vi "Dashboard Main.vi"() -> ()   [LabVIEW 2016]
uses:
  <vilib>/Rock Robotics/WPI/Camera/WPI_CameraExposure Values.ctl
  <vilib>/Rock Robotics/WPI/Camera/WPI_CameraWhite Balance Values.ctl
  <vilib>/Rock Robotics/WPI/Camera/WPI_CameraSettings Read MJPG.ctl
  <vilib>/Rock Robotics/WPI/Camera/WPI_CameraImageSize.ctl
  <vilib>/Utility/miscctls.llb/LVRowAndColumnTypeDef.ctl
  <vilib>/event_ctls.llb/eventvkey.ctl
  <vilib>/Rock Robotics/Network Tables/NT Read Numeric Array.vi
  <vilib>/Rock Robotics/Network Tables/NT Write Boolean.vi
  <vilib>/Rock Robotics/WPI/Dashboard/WPI_DashboardLogging Global.vi
  <vilib>/vision/NI_Vision_Development_Module.lvlib
panel:
  in  "Camera Settings Right":T1={"Frame Rate"=30, "Compression"=30, "Size"=1, "DB Camera Config"=FALSE} {"Frame Rate" scale=1.0..30.0; "Compression" scale=100.0..-1.0; "Size" items=["640x480", "320x240", "160x120"]}
  in  "Camera Name Right":string(combo)="No Camera Selection"
  out "Camera Info":cluster{"Mbps LED":bool, "Mbps":dbl, "fps":dbl} {"fps" format="%#.1g"; "Mbps" format="%#.1g"}
  in  "Camera Settings":T1={"Frame Rate"=30, "Compression"=30, "Size"=1, "DB Camera Config"=FALSE} {"Frame Rate" scale=1.0..30.0; "Compression" scale=100.0..-1.0; "Size" items=["640x480", "320x240", "160x120"]}
  in  "TCP":refnum<k5>
  in  "Rec Mode":enum32{"Stop", "Record", "Playback"}(radio)
  out "Robot IP":string
  out "Image Message":string="Timeout in Camera Communications"
  in  "Dashboard Tab":T2(tab)
  in  "New Gyro":bool
  in  "Degrees Rotated":dbl
  in  "NumAcq":dbl
  in  "Forward Time":dbl
  in  "Station":enum16{"1", "2", "3"}(ring)
  in  "OVERRIDE":bool
  in  "Offset":dbl
  out "Reverse":bool
  in  "Degree  Error":dbl=2.0
  in  "Acq Boundary":dbl=15.0
  in  "Target Drive Speed":dbl=-0.5
  in  "Target Pivot Speed":dbl=0.48
  in  "Comp Bot?":bool
  out "Error Value":dbl
  in  "Left Station":bool caption="Left Station?"
  in  "Select Auto":string(combo)="Your Turn"
  out "NT Connection":bool
  out "MotorChart R":cluster{"Numeric":dbl, "Numeric":dbl}(graph)
  out "MotorChart L":cluster{"Numeric":dbl, "Numeric":dbl}(graph)
  out "MotorSliders R":cluster{"MotorSlide1":dbl, "MotorSlide2":dbl} {"MotorSlide2" scale=-1.0..1.0 scale format="%#_2e"; "MotorSlide1" scale=-1.0..1.0 scale format="%#_2e"}
  out "MotorSliders L":cluster{"MotorSlide1":dbl, "MotorSlide2":dbl} {"MotorSlide2" scale=-1.0..1.0 scale format="%#_2e"; "MotorSlide1" scale=-1.0..1.0 scale format="%#_2e"}
  out "Gyro":dbl(knob) scale=0.0..360.0
  out "JS1 Z":dbl(slide) scale=-1.0..1.0 scale format="%#_2e"
  out "JS1 Graph":cluster{"X":dbl, "Y":dbl}[](graph)
  out "JS1 Buttons":T3
  out "JS2 Z":dbl(slide) scale=-1.0..1.0 scale format="%#_2e"
  out "JS2 Graph":cluster{"X":dbl, "Y":dbl}[](graph)
  out "JS2 Buttons":T3
  out "Mode":T4(ring)=enum."Auto Disabled"
  out "Camera Active":bool
  out "Camera Image Right":T5(plugin-control)
  in  "DB/String 9":string
  in  "DB/String 8":string
  in  "DB/String 7":string
  in  "DB/String 6":string
  in  "DB/String 5":string
  in  "DB/String 4":string
  in  "DB/String 3":string
  in  "DB/String 2":string
  in  "DB/String 1":string
  in  "DB/String 0":string
  in  "DB/Slider 0":dbl(slide) scale=0.0..5.0
  in  "DB/Slider 1":dbl(slide) scale=0.0..5.0
  in  "DB/Slider 2":dbl(slide) scale=0.0..5.0
  in  "DB/Slider 3":dbl(slide) scale=0.0..5.0
  out "DB/LED 3":bool
  out "DB/LED 2":bool
  out "DB/LED 1":bool
  out "DB/LED 0":bool
  in  "DB/Button 3":bool
  in  "DB/Button 2":bool
  in  "DB/Button 1":bool
  in  "DB/Button 0":bool caption="New Name"
  out "String":string
  in  "Test Slider":dbl(slide) scale=0.0..100.0 scale format="%#_3g"
  in  "On/Off":bool caption="Solenoid"
  in  "Test Name":u16(ring) items=["Select the test to run..."]
  in  "Test Tree":string(tree)
  in  "Motor":cluster{"Value":dbl, "Enable":bool} {"Value" scale=-1.0..1.0 scale format="%#_3g"}
  out "Progress":T6 {"Test Progress" scale=0.0..100.0}
  in  "Rev/Fwd":cluster{"Forward":bool, "Reverse":bool}
  in  "Test Ring":u16(ring) items=["Monochrome", "Color"]
  out "Cmd Status":string
  in  "Execute Command":bool
  in  "Command Params":string[][](table)
  in  "Command Selection":i32(listbox)
  in  "CheckList":i32(listbox)
  out "Tree":string(tree)
  out "Camera Image":T5(plugin-control)
  out "Background":bool
  in  "Camera Name":string(combo)="No Camera Selection"
  # "HW"
  # "HW"
  # "Joysticks"
  # "Drive Motors"
  # "Front"
  # "Right"
  # "Left"
  # "Back"
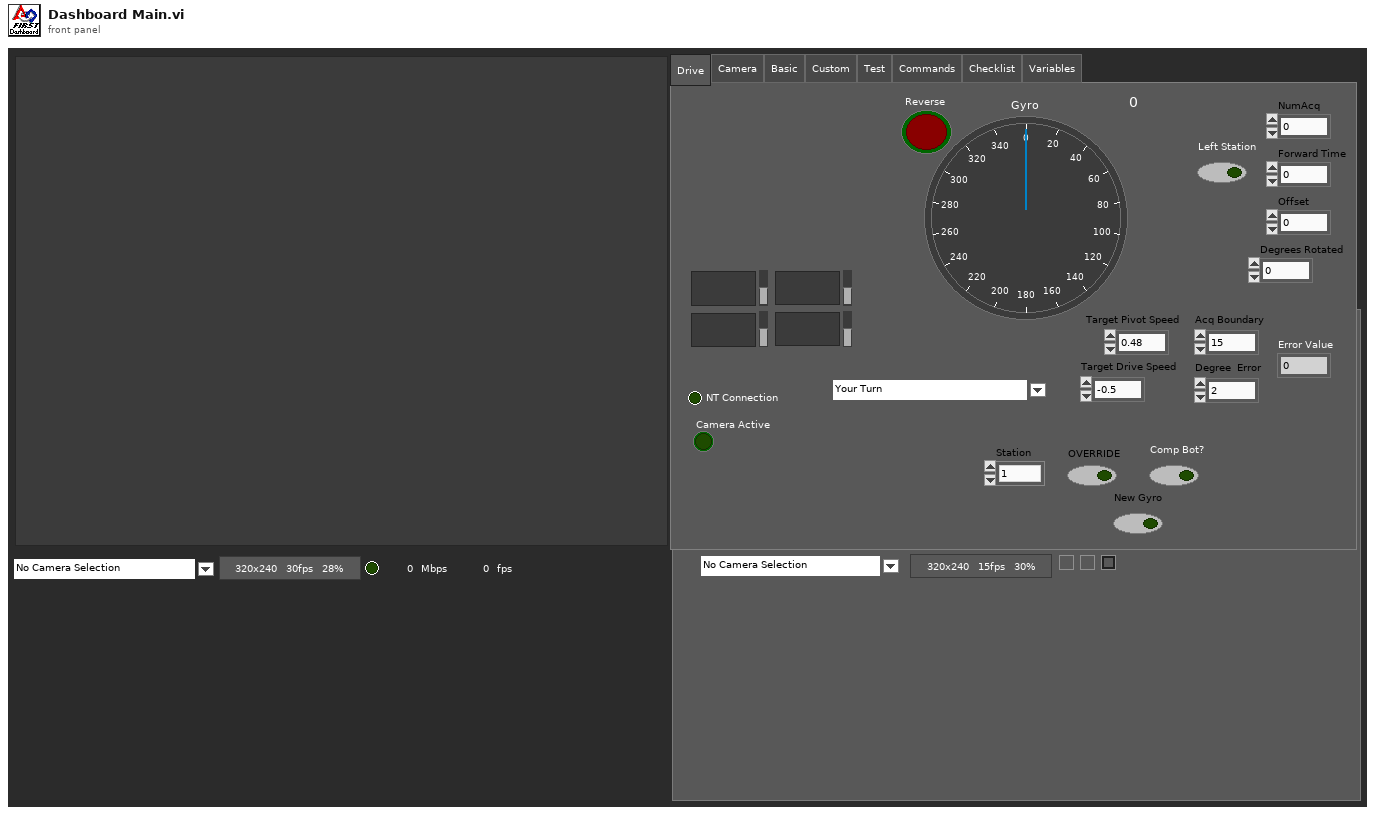
[diagram p1: front panel]
types:
  T1 = cluster{"Frame Rate":i32, "Compression":i32, "Size":u16, "DB Camera Config":bool}
  T2 = enum32{"Drive", "Camera", "Basic", "Custom", "Test", "Commands", "Checklist", "Variables"}
  T3 = cluster{bool, bool, bool, bool, bool, bool, bool, bool, bool, bool, bool, bool}
  T4 = enum8{"Tele-Op Disabled", "Tele-Op Enabled", "Auto Disabled", "Auto Enabled", "Test Disabled", "Test Enabled", "Disconnected", "No Code", "E-Stop"}
  T5 = typedef "IMAQ Image.ctl" = refnum<image>
  T6 = cluster{"Test Progress":u8, "Test Progress Text":string}
  T7 = typedef "Image Type" = u32
  T8 = cluster{"IDs":cluster{"RPC field ID":u16, "Unique ID":u16}, "String":string}
  T9 = enum32{"Drive", "Basic", "Custom", "Test", "Checklist", "Variables"}
  T10 = typedef "WPI_CameraSettings Read MJPG.ctl" = cluster{"fps":i32, "compression":i32, "Image Size":T11, "Config Shown":bool}
  T11 = typedef "WPI_CameraImageSize.ctl" = enum16{"640x480", "320x240", "160x120", "Custom"}
  T12 = typedef "WPI_CameraExposure Values.ctl" = enum16{"Auto", "Flicker-free 50 Hz", "Flicker-free 60 Hz", "Hold current", "Custom"}
  T13 = typedef "WPI_CameraWhite Balance Values.ctl" = enum16{"Auto", "Fixed indoor", "Fixed outdoor 1", "Fixed outdoor 2", "Fixed fluorescent 1", "Fixed fluorescent 2", "Hold current", "Custom"}
  T14 = cluster{"Exposure":T12, "Exposure (%)":dbl, "Brightness":i32, "White Balance":T13, "Color Temp (K)":dbl}
  T15 = cluster{"Brightness":sgl, "Contrast":sgl, "Gamma":sgl}
  T16 = cluster{"Camera Image":refnum<vi>, "Dashboard Tab":refnum<vi>, "Background":refnum<vi>, "Rec Mode":refnum<vi>, "Test Slider":refnum<vi>, "On/Off ":refnum<vi>, "Test Ring":refnum<vi>, "Rev/Fwd":refnum<vi>, "Test Name":refnum<vi>, "Motor":refnum<vi>, "Progress":refnum<vi>, "CheckList":refnum<vi>, "Tree":refnum<vi>, "Test Tree":refnum<vi>, "Command Params":refnum<vi>, "Command Selection":refnum<vi>, "Execute Command":refnum<vi>, "Cmd Status":refnum<vi>, "Camera Settings":refnum<vi>, "Camera Name":refnum<vi>, "Camera Info":refnum<vi>, "Camera Settings Right":refnum<vi>, "Camera Name Right":refnum<vi>, "Camera Image Right":refnum<vi>}
  T17 = cluster{"Error Strings":string, "Disable Counts":cluster{u16, u16}, "Rail Faults":cluster{u16, u16, u16}, "Robot IP":string, "DB Mode":u8, "Event Info":cluster{"Name":string, "Type":u8, "Number":u16, "Replay":u8}}
  T18 = cluster{"Storage":cluster{"Disk Free":u64, "RAM Block":u32, "RAM free":u32}, "CPU Utilization":cluster{"CPU % ISR":sgl, "CPU % Time Crit":sgl, "CPU % Timed Str":sgl, "CPU % High":sgl, "CPU % Above":sgl, "CPU % Normal":sgl, "CPU % Low":sgl}, "CAN":cluster{"% Bus Utilization":sgl, "Bus Off Cnt":u32, "TX_FIFO Full Cnt":u32, "Receive Error Cnt":u8, "Transmit Error Cnt":u8}, "HID":cluster{"HID Outputs":u32, "Rumble Low":u16, "Rumble High":u16}[]}
  T19 = cluster{"Status bits":cluster{"Test Mode":bool, "Autonomous":bool, "Enabled":bool, "Code Start":bool, "Brownout":bool, "Reserved 2":bool, "Reserved 3":bool, "E-Stop":bool}, "Code Trace":cluster{"Disabled":bool, "TeleOp":bool, "Auto":bool, "Test":bool}, "Controller Type":enum16{"unknown", "cRIO", "roboRio"}, "Code?":enum16{"unknown", "noCode", "code"}, "Battery V":dbl}
  T20 = cluster{"Control Bits":cluster{"TestMode":bool, "Autonomous":bool, "Enabled":bool, "FMS Present":bool, bool, bool, bool, "E-Stop":bool}, "Team Station ":u8, "Countdown":sgl, "Joystick Values":cluster{"Axes":dbl[], "Buttons":bool[], "POVs":i16[]}[]}
  T21 = cluster{"Axes":dbl[], "Buttons":bool[], "POVs":i16[]}[]
  T22 = cluster{"Axes":dbl[], "Buttons":bool[], "POVs":i16[]}
  T23 = cluster{"Buttons[0]":bool, "Buttons[1]":bool, "Buttons[2]":bool, "Buttons[3]":bool, "Buttons[4]":bool, "Buttons[5]":bool, "Buttons[6]":bool, "Buttons[7]":bool, "Buttons[8]":bool, "Buttons[9]":bool, "Buttons[10]":bool, "Buttons[11]":bool}
  T24 = cluster{"Operation":enum16{"Update", "Clear"}, "Color Box":u32}[]
  T25 = typedef "eventvkey.ctl" = enum16{"ASCII", "Enter", "Return", "Shift", "Ctrl", "Alt", "Cmd", "Opt", "Caps", "NumLock", "Clear", "Break", "Up", "Down", "Left", "Right", "Insert", "Delete", "Home", "End", "PageUp", "PageDown", "Escape", "Help", "Pause", "ScrollLock", "F1", "F2", "F3", "F4", "F5", "F6", "F7", "F8", "F9", "F10", "F11", "F12", "F13", "F14", "F15", "F16", "F17", "F18", "F19", "F20", "F21", "F22", "F23", "F24", "Play", "VolumeUp", "VolumeDown", "Mute", "Two Byte Char"}
  T26 = cluster{"Image Size":bool, "Image Type":bool, "Pixel Value":bool, "ROI Information":bool, "Zoom Factor":bool}
  T27 = cluster{"Operation":enum16{"Update", "Clear"}, "Color Box":u32}
  T28 = typedef "LVRowAndColumnTypeDef.ctl" = cluster{"Row":i32, "Column":i32}
  T29 = cluster{"Shift":bool, "Ctrl":bool, "Alt":bool, "Cmd":bool, "Opt":bool}
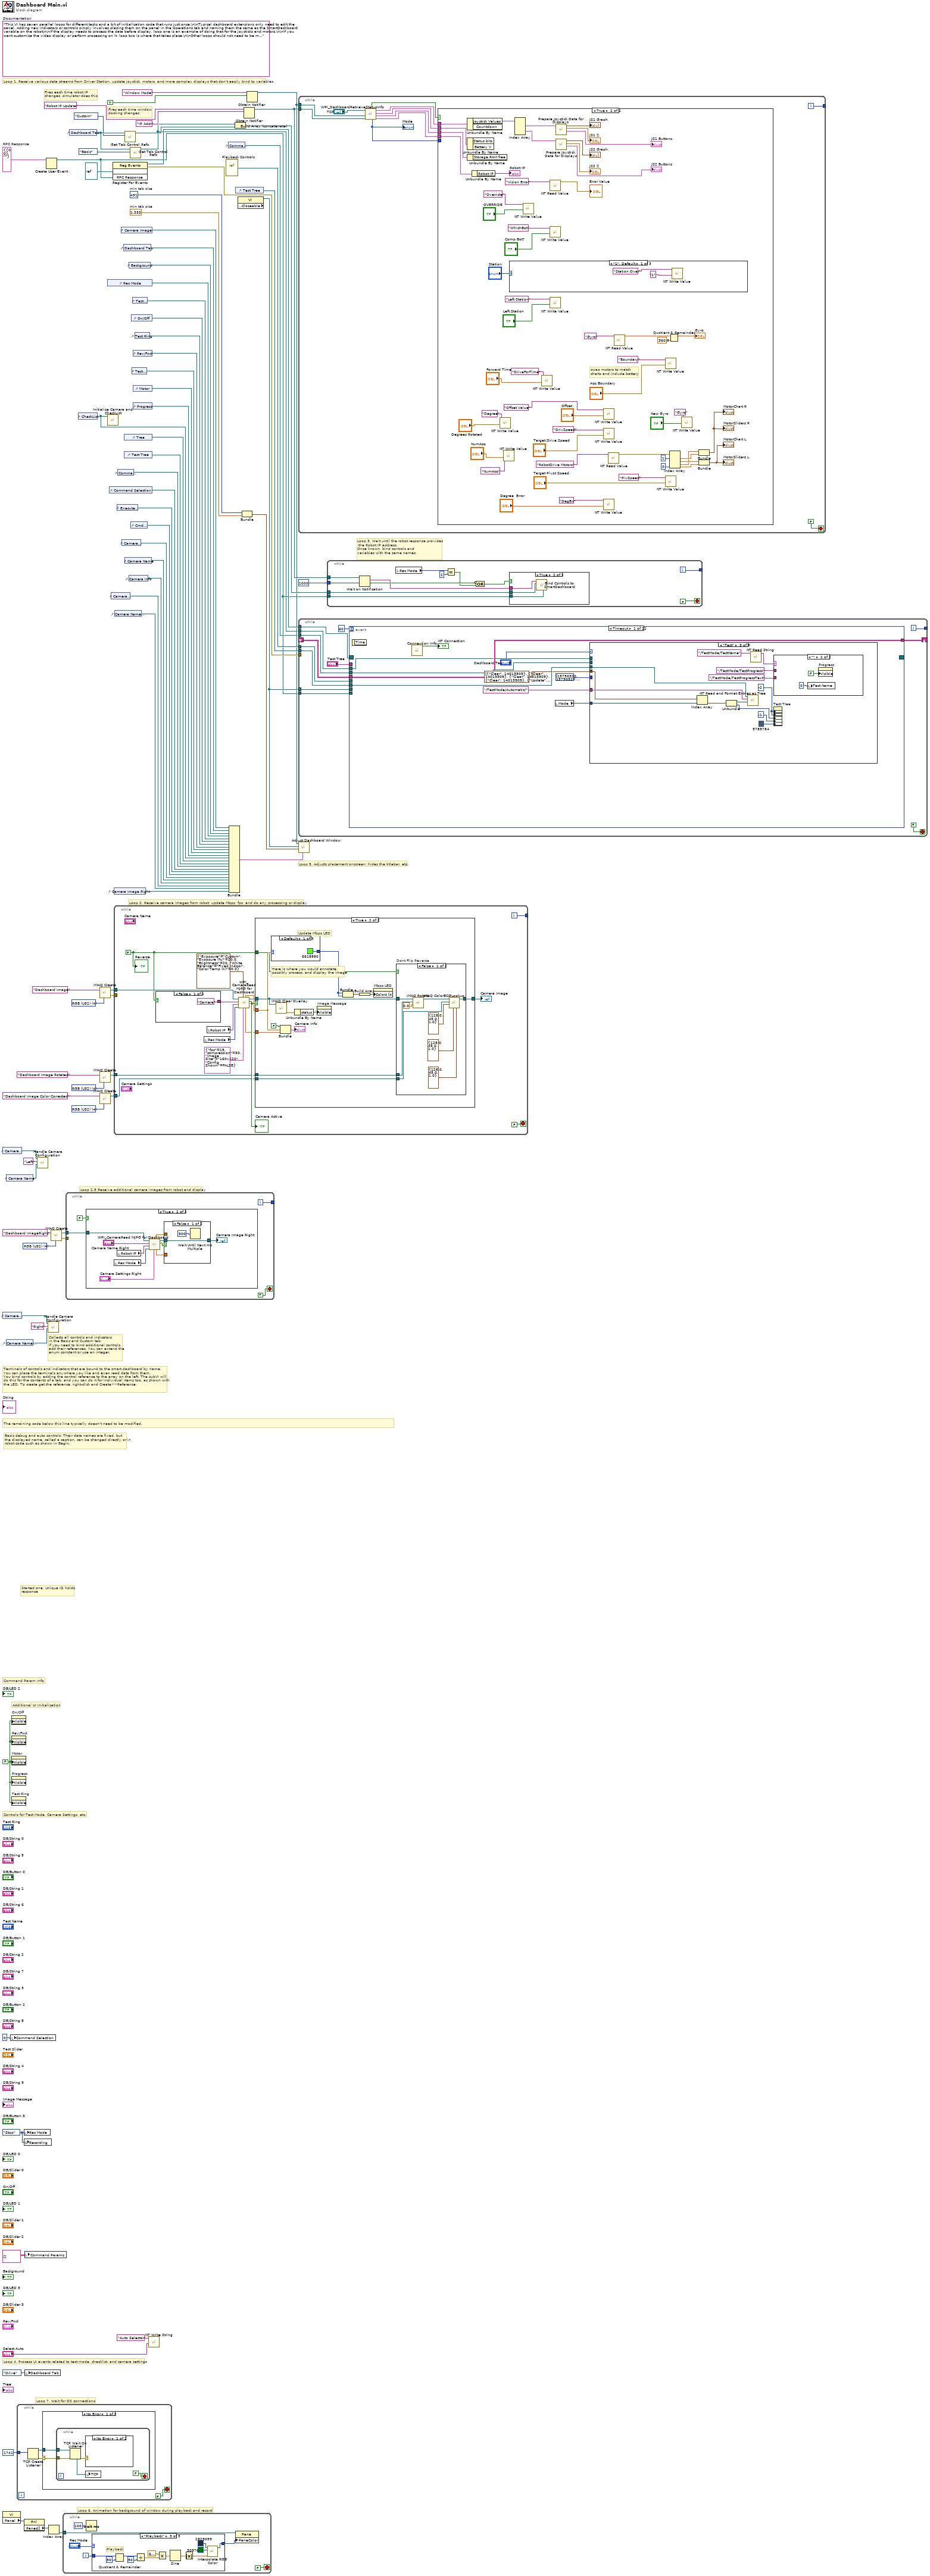
[diagram p0: block diagram]
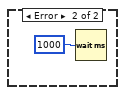
[diagram p4: hidden frame]
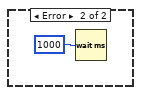
[diagram p5: hidden frame]
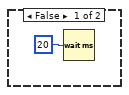
[diagram p6: hidden frame]
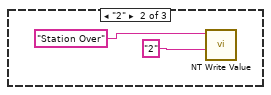
[diagram p7: hidden frame]
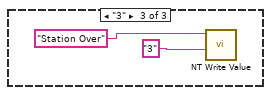
[diagram p8: hidden frame]
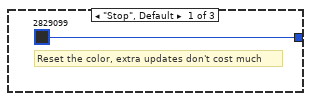
[diagram p9: hidden frame]
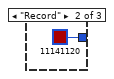
[diagram p10: hidden frame]
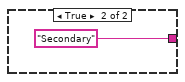
[diagram p12: hidden frame]
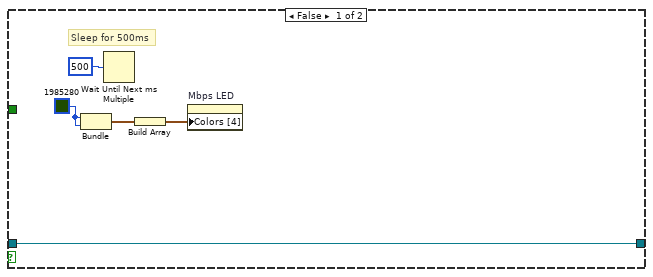
[diagram p13: hidden frame]
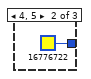
[diagram p15: hidden frame]
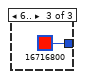
[diagram p16: hidden frame]
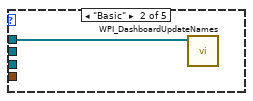
[diagram p18: hidden frame]
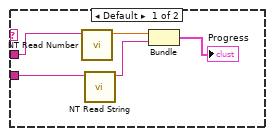
[diagram p19: hidden frame]
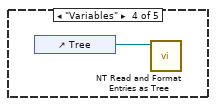
[diagram p20: hidden frame]
diagram:
  w3 = T7 4 items=["Grayscale (U8)", "Grayscale (I16)", "Grayscale (SGL)", "Complex (CSG)", "RGB (U32)", "HSL (U32)", "RGB (U64)"] ("Image Type")
  w6 = T7 4 items=["Grayscale (U8)", "Grayscale (I16)", "Grayscale (SGL)", "Complex (CSG)", "RGB (U32)", "HSL (U32)", "RGB (U64)"] ("Image Type")
  w16 = T7 4 items=["Grayscale (U8)", "Grayscale (I16)", "Grayscale (SGL)", "Complex (CSG)", "RGB (U32)", "HSL (U32)", "RGB (U64)"] ("Image Type")
  w32 = T8 {"IDs"={"RPC field ID"=0, "Unique ID"=0}, "String"=""}  # RPC Response
  w57 = 491  # min tab size
  w56 = 1.333  # min tab size
  w64 = enum32{"Stop", "Record", "Playback"}."Stop" ("Rec Mode")
  w39 = FALSE ("Visible")
  (unwired) "This VI has seven parallel loops for different tasks and a bit of initialization code that runs just once.\n\nTypical dashboard extensions only need to edit the panel. Adding new indicators or controls simply involves placing them on the panel in the Operations tab and naming them the same as the SmartDashboard variable on the robot\n\nIf the display needs to process the data before display, loop one is an example of doing that for the joysticks and motors.\n\nIf you want customize the video display or perform processing on it, loop two is where that takes place.\n\nOther loops should not need to be modified. They are pretty standard, and document the task they perform."  # Documentation
  w81 = T7 4 items=["Grayscale (U8)", "Grayscale (I16)", "Grayscale (SGL)", "Complex (CSG)", "RGB (U32)", "HSL (U32)", "RGB (U64)"] ("Image Type")
  # "Loop 2.5 Receive additional camera images from robot and display"
  # "Command Param Info"
  # "Started one, Unique ID holds\nresponse"
  # "Loop 7. Wait for DS connections"
  # "Basic debug and auto controls: Their data names are fixed, but\nthe displayed name, called a caption, can be changed directly or in\nrobot code such as shown in Begin."
  # "Controls for Test Mode, Camera Settings, etc."
  # "Additional UI Initialization"
  # "Loop 6. Animation for background of window during playback and record"
  # "Fires each time robot IP\nchanges, simulator does this"
  # "Fires each time window\ndocking changes."
  # "Collects all controls and indicators\nin the Basic and Custom tab.\nIf you need to bind additional controls,\nadd their references. You can extend the\nenum constant or use an integer."
  # "The remaining code below this line typically doesn't need to be modified."
  # "Loop 4. Process UI events related to test mode, checklist, and camera settings"
  # "Terminals of controls and indicators that are bound to the smart dashboard by name.\nYou can place the terminals anywhere you like and even read data from them.\nYou bind controls by adding the control reference to the array on the left. The subVI will\ndo this for the contents of a tab, and you can do it for individual items too, as shown with\nthe LED. To create get the reference, right-click and Create>>Reference."
  # "Loop 3. Wait until the robot response provides\n the Robot IP address.\nOnce known, bind controls and\nvariables with the same names."
  # "Loop 5. Adjusts placement onscreen, hides the titlebar, etc."
  # "Loop 1. Receive various data streams from Driver Station, update joystick, motors, and more complex displays that don't easily bind to variables."
  # "Loop 2. Receive camera images from robot, update Mbps, fps, and do any processing or display"
  n1 = control-ref of="Camera Settings"() -> (w25:refnum<vi>)
  n2 = control-ref of="Camera Settings Right"() -> (w13:refnum<vi>)
  n3 = property class="VI"() -> ("Panel"=w71:refnum<vi>)  [unwired: 2 in, 2 out]
  n4 = control-ref of="Camera Name"() -> (w24:refnum<vi>)
  n5 = control-ref of="Camera Name Right"() -> (w12:refnum<vi>)
  n6 = local write "Command Selection"(u16 0 ("milliseconds to wait")) -> ()
  n7 = property on="On/Off" class="Bool (strict)"("Visible"=w39) -> ()  [unwired: 2 in, 2 out]
  n8 = property on="Rev/Fwd" class="Clust (strict)"("Visible"=w39) -> ()  [unwired: 2 in, 2 out]
  n9 = property on="Motor" class="Clust (strict)"("Visible"=w39) -> ()  [unwired: 2 in, 2 out]
  n10 = property on="Progress" class="Clust (strict)"("Visible"=w39) -> ()  [unwired: 2 in, 2 out]
  n11 = property on="Test Ring" class="Ring (strict)"("Visible"=w39) -> ()  [unwired: 2 in, 2 out]
  n12 = while {
    tunnel: u16 1741 ("timeout ms (25000)") -> [w83]
    stop <- FALSE stop-if-true
    n13 = TCP Create Listener(10:w83) -> (0:w82:errorcluster, 3:w84:refnum<k5>)  [unwired: 4 in, 1 out]
    n14 = case shown="No Error" w82 {
      selector: w82 -> [w86 _]
      tunnel: w84 -> [w87 _]
      frame No Error {
        n15 = while {
          tunnel: w87 -> [w90]
          tunnel: w86 -> [w89]
          stop <- FALSE stop-if-true
          n16 = TCP Wait On Listener(8:w89, 11:w90) -> (0:w91:errorcluster, 4:w92:refnum<k5>)  [unwired: 2 in, 3 out]
          n17 = case shown="No Error" w91 {
            frame No Error {
            }
            frame Error {
              n18 = Wait (ms)(milliseconds to wait=u32 1000) -> ()  [unwired: 1 out]
            }
          }
          n19 = local write "TCP"(w92) -> ()
        }
      }
      frame Error {
        n20 = Wait (ms)(milliseconds to wait=u32 1000) -> ()  [unwired: 1 out]
      }
    }
  }
  n21 = local write "Rec Mode"(w64) -> ()
  n22 = global write "WPI_DashboardLogging Global.vi" "Recording"(w64) -> ()
  n23 = property class="Pnl"(reference=w71) -> ("Panes[]"=w72:refnum<vi>[])  [unwired: 1 in, 2 out]
  n24 = local write "Command Params"(string[][] [] ("Command Params")) -> ()
  n25 = local write "Dashboard Tab"(T2."Drive" ("Dashboard Tab")) -> ()
  n26 = call "Handle Camera Configuration.vi"("CameraNameRef"=w24, "Camera File Name"="Left", "ClusterRef"=w25) -> ()  [unwired: 9 in]
  n27 = Create User Event(user event datatype=w32) -> (user event=w28:refnum<user-event>)  [unwired: 1 in, 1 out]
  n28 = call "Handle Camera Configuration.vi"("CameraNameRef"=w12, "Camera File Name"="Right", "ClusterRef"=w13) -> ()  [unwired: 9 in]
  n29 = Index Array(array=w72) -> (element=w70:refnum<vi>)  [unwired: 1 in]
  n30 = call "IMAQ Create"("Image Name"="Dashboard ImageRight", "Image Type"=w16) -> ("New Image"=w15:T5, "error out"=w14:errorcluster)  [unwired: 2 in, 1 out]
  n31 = while {
    tunnel: w70 -> [w96]
    i -> [w99]
    stop <- FALSE stop-if-true
    n32 = Wait (ms)(milliseconds to wait=u32 100) -> ()  [unwired: 1 out]
    n33 = case shown="\"Playback\"" "Rec Mode" {
      tunnel: w99 -> [_ _ w114]
      tunnel: [u32 2829099 ("Base Color") u32 11141120 ("Target Color") w103] -> w95
      frame "Stop", Default {
        # "Reset the color, extra updates don't cost much"
      }
      frame "Record" {
      }
      frame "Playback" {
        # "Playback"
        n34 = Quotient & Remainder(x=w114, y=u32 50 ("milliseconds to wait")) -> (x-y*floor(x/y)=w110:u32)  [unwired: 1 out]
        n35 = Divide(x=w110, y=u32 50 ("milliseconds to wait")) -> (x/y=w107:dbl)
        n36 = Multiply(x=6.283185307179586, y=w107) -> (x*y=w112:dbl)
        n37 = Sine(x=w112) -> (sin(x)=w111:dbl)
        n38 = Absolute Value(x=w111) -> (abs(x)=w104:dbl)
        n39 = call "Interpolate RGB Color.vi"("Proportion"=w104, "Target Color"=u32 30976, "Base Color"=u32 2829099) -> ("Result Color"=w103:u32)  [unwired: 8 in]
      }
    }
    n40 = property class="Pane"(reference=w96, "PaneColor"=w95) -> ()  [unwired: 1 in, 2 out]
  }
  n41 = while {
    tunnel: w15 -> [w118]
    tunnel: w14 -> [_]
    tunnel: [w117] -> _
    i -> [w117]
    stop <- TRUE stop-if-true
    n42 = case shown="True" FALSE {
      tunnel: w118 -> [_ w127]
      frame False {
      }
      frame True {
        n43 = local read "Rec Mode"() -> (w125:enum32{"Stop", "Record", "Playback"})
        n44 = local read "Robot IP"() -> (w126:string)
        n45 = call <vilib>:"WPI_CameraRead MJPG for Dashboard.vi"("Camera Settings"="Camera Settings Right", "Rec Mode"=w125, "Robot IP"=w126, "Camera Name"="Camera Name Right", "Refnum in"=w127) -> ("Active"=w122:bool, "Refnum out"=w123:T5, "FPS"=w120:dbl, "Bandwidth (Mbps)"=w121:dbl)  [unwired: 3 in]
        n46 = case shown="False" w122 {
          tunnel: w123 -> [w129 w131]
          tunnel: w121 -> [_ _]
          tunnel: w120 -> [_ _]
          tunnel: [w129 w131] -> w119
          frame False {
            n47 = Wait Until Next ms Multiple(millisecond multiple=u32 500) -> ()  [unwired: 1 out]
          }
          frame True {
          }
        }
        "Camera Image Right" <- w119
      }
    }
  }
  n48 = control-ref of="Dashboard Tab"() -> (w62:refnum<vi>)
  n49 = control-ref of="CheckList"() -> (w50:refnum<vi>)
  n50 = call "IMAQ Create"("Image Name"="Dashboard Image", "Image Type"=w81) -> ("New Image"=w79:T5, "error out"=w78:errorcluster)  [unwired: 2 in, 1 out]
  n51 = call "IMAQ Create"("Image Name"="Dashboard Image Rotated", "Image Type"=w6) -> ("New Image"=w4:T5)  [unwired: 2 in, 2 out]
  n52 = call "IMAQ Create"("Image Name"="Dashboard Image Color Corrected", "Image Type"=w3) -> ("New Image"=w1:T5)  [unwired: 2 in, 2 out]
  n53 = control-ref of="Rec Mode"() -> (w45:refnum<vi>)
  n54 = call "Initialize Camera and CheckList.vi"("ListBox in"=w50) -> ()  [unwired: 11 in]
  n55 = control-ref of="Command Selection"() -> (w31:refnum<vi>)
  n56 = control-ref of="Camera Settings Right"() -> (w9:refnum<vi>)
  n57 = register-events(refnum<vi> refnum, w28) -> (reference out=w68:refnum<event-registration>, error out=w67:errorcluster)  [unwired: 2 in]
  n58 = control-ref of="Camera Image Right"() -> (w7:refnum<vi>)
  n59 = while {
    tunnel: w79 -> [w145]
    tunnel: w78 -> [_]
    tunnel: [w146] -> _
    tunnel: w4 -> [w137]
    tunnel: w1 -> [w136]
    i -> [w146]
    stop <- FALSE stop-if-true
    w132 = FALSE ("Default Value")
    n60 = case shown="False" w132 {
      tunnel: ["Camera" "Secondary"] -> w135
      frame False {
      }
      frame True {
      }
    }
    n61 = local read "Rec Mode"() -> (w141:enum32{"Stop", "Record", "Playback"})
    n62 = local read "Robot IP"() -> (w140:string)
    n63 = call <vilib>:"WPI_CameraRead MJPG for Dashboard.vi"("Camera Settings"=T10 {"fps"=15, "compression"=30, "Image Size"=enum."160x120", "Config Shown"=FALSE}, "Camera Settings 2"=T14 {"Exposure"=enum."Custom", "Exposure (%)"=20.0, "Brightness"=20, "White Balance"=enum."Fixed indoor", "Color Temp (K)"=0.0}, "Rec Mode"=w141, "Robot IP"=w140, "Camera Name"=w135, "Refnum in"=w145) -> ("Active"=w143:bool, "Refnum out"=w144:T5, "FPS"=w142:dbl, "Bandwidth (Mbps)"=w139:dbl)  [unwired: 2 in]
    "Camera Active" <- w143
    n64 = case shown="True" w143 {
      tunnel: w144 -> [w150 w159]
      tunnel: w139 -> [_ w162]
      tunnel: w142 -> [_ w163]
      tunnel: [w150 w155] -> w138
      tunnel: w137 -> [_ w158]
      tunnel: w136 -> [_ w156]
      tunnel: w132 -> [_ w157]
      frame False {
        w152 = u32 1985280 ("Color Box")
        # "Sleep for 500ms"
        n65 = Bundle("Color Box"=w152, "Color Box"=w152) -> (w153:cluster{"Color Box":u32, "Color Box":u32})  [unwired: 1 out]
        n66 = Wait Until Next ms Multiple(millisecond multiple=u32 500) -> ()  [unwired: 1 out]
        n67 = Build Array(w153) -> (w151:cluster{"Color Box":u32, "Color Box":u32}[])
        n68 = property on="Mbps LED" class="Bool (strict)"("Colors [4]"=w151) -> ()  [unwired: 2 in, 2 out]
      }
      frame True {
        # "Here is where you would annotate,\npossibly process, and display the image"
        # "Update Mbps LED"
        n69 = case shown="Default" w162 {
          tunnel: [u32 6618880 ("Color Box") u32 16776722 ("Color Box") u32 16716800 ("Color Box")] -> w165
          frame Default {
          }
          frame 4, 5 {
          }
          frame 6.. {
          }
        }
        n70 = call "IMAQ Clear Overlay"("Image"=w159) -> ("error out"=w167:errorcluster)  [unwired: 2 in, 8 out]
        n71 = Bundle(FALSE, "Bandwidth (Mbps)"=w162, "FPS"=w163) -> (→"Camera Info":cluster{bool, "Bandwidth (Mbps)":dbl, "FPS":dbl})  [unwired: 1 in]
        n72 = Unbundle By Name(w167) -> ("status"=w168:bool)
        n73 = property on="Image Message" class="Str"("Visible"=w168) -> ()  [unwired: 2 in, 2 out]
        n74 = Bundle("Color Box"=w165, "Color Box"=w165) -> (w166:cluster{"Color Box":u32, "Color Box":u32})  [unwired: 1 out]
        n75 = Build Array(w166) -> (w164:cluster{"Color Box":u32, "Color Box":u32}[])
        n76 = property on="Mbps LED" class="Bool (strict)"("Colors [4]"=w164) -> ()  [unwired: 2 in, 2 out]
        n77 = case "Dont Flip Reverse" shown="False" w157 {
          tunnel: w159 -> [w176 w178]
          tunnel: w158 -> [w175 _]
          tunnel: w156 -> [w171 _]
          tunnel: [w169 w178] -> w155
          frame False {
            n78 = call "IMAQ Rotate"("Angle (degrees)"=sgl 0.0, "Image Dst"=w175, "Image Src"=w176) -> ("Image Dst Out"=w170:T5)  [unwired: 7 in, 1 out]
            n79 = call "IMAQ ColorBCGLookup"("Blue BCG Values"=T15 {"Brightness"=128.0, "Contrast"=45.0, "Gamma"=1.0}, "Green BCG Values"=T15 {"Brightness"=128.0, "Contrast"=45.0, "Gamma"=1.0}, "Red BCG Values"=T15 {"Brightness"=128.0, "Contrast"=45.0, "Gamma"=1.0}, "Image Dst"=w171, "Image Src"=w170) -> ("Image Dst Out"=w169:T5)  [unwired: 5 in, 1 out]
          }
          frame True {
          }
        }
      }
    }
    "Camera Image" <- w138
    "Reverse" <- w132
  }
  n80 = control-ref of="Camera Name Right"() -> (w8:refnum<vi>)
  n81 = control-ref of="Execute Command"() -> (w33:refnum<vi>)
  n82 = control-ref of="Command Params"() -> (w34:refnum<vi>)
  n83 = control-ref of="Camera Image"() -> (w59:refnum<vi>)
  n84 = control-ref of="Camera Settings"() -> (w23:refnum<vi>)
  n85 = control-ref of="Dashboard Tab"() -> (w58:refnum<vi>)
  n86 = control-ref of="Tree"() -> (w49:refnum<vi>)
  n87 = control-ref of="Test Tree"() -> (w48:refnum<vi>)
  n88 = call <vilib>:"Get Tab Control Refs.vi"("Page Index"=T9."Custom" ("Dashboard Tab"), "TabControl in"=w62) -> ("ControlsOnPage"=w61:refnum<vi>[])  [unwired: 9 in]
  n89 = control-ref of="Camera Name"() -> (w22:refnum<vi>)
  n90 = control-ref of="Background"() -> (w54:refnum<vi>)
  n91 = control-ref of="Camera Info"() -> (w21:refnum<vi>)
  n92 = call <vilib>:"Get Tab Control Refs.vi"("Page Index"=T9."Basic" ("Dashboard Tab"), "TabControl in"=w62) -> ("ControlsOnPage"=w20:refnum<vi>[])  [unwired: 9 in]
  n93 = control-ref of="Cmd Status"() -> (w27:refnum<vi>)
  n94 = control-ref of="On/Off"() -> (w43:refnum<vi>)
  n95 = control-ref of="Test Name"() -> (w47:refnum<vi>)
  n96 = control-ref of="Test Slider"() -> (w44:refnum<vi>)
  n97 = control-ref of="Rev/Fwd"() -> (w41:refnum<vi>)
  n98 = control-ref of="Motor"() -> (w46:refnum<vi>)
  n99 = control-ref of="Progress"() -> (w40:refnum<vi>)
  n100 = control-ref of="Test Ring"() -> (w42:refnum<vi>)
  n101 = call <vilib>:"NT Write String.vi"("String"="Select Auto", "Name"="Auto Selector") -> ()  [unwired: 9 in, 1 out]
  n102 = vi-ref "Playback Controls.vi"() -> (w69:refnum<vi>)
  n103 = control-ref of="Command Params"() -> (w26:refnum<vi>)
  n104 = Bundle("Camera Image"=w59, "Dashboard Tab"=w58, "Background"=w54, "Rec Mode"=w45, "Test Slider"=w44, "On/Off"=w43, "Test Ring"=w42, "Rev/Fwd"=w41, "Test Name"=w47, "Motor"=w46, "Progress"=w40, "CheckList"=w50, "Tree"=w49, "Test Tree"=w48, "Command Params"=w34, "Command Selection"=w31, "Execute Command"=w33, "Cmd Status"=w27, "Camera Settings"=w23, "Camera Name"=w22, "Camera Info"=w21, "Camera Settings Right"=w9, "Camera Name Right"=w8, "Camera Image Right"=w7) -> (w51:T16)  [unwired: 1 in]
  n105 = Build Array (concatenate)(w20, w61) -> (w60:refnum<vi>[])
  n106 = control-ref of="Test Tree"() -> (w73:refnum<vi>)
  n107 = property class="VI" props=["Front Panel.Closeable"]() -> (reference out=w63:refnum<vi>)  [unwired: 2 in, 2 out]
  n108 = Bundle("min tab size"=w57, "min tab size"=w56) -> (w55:cluster{"min tab size":i32, "min tab size":dbl})  [unwired: 1 in]
  n109 = Obtain Notifier(name (unnamed)="Robot IP Update", notification data type="IP Addr" ("name (unnamed)")) -> (notifier out=w38:refnum<notifier>)  [unwired: 2 in, 2 out]
  n110 = Obtain Notifier(name (unnamed)="Window Mode", notification data type=TRUE) -> (notifier out=w37:refnum<notifier>)  [unwired: 2 in, 2 out]
  n111 = while {
    tunnel: [w191] -> _
    tunnel: w38 -> [w185]
    tunnel: w37 -> [w182]
    i -> [w191]
    stop <- FALSE stop-if-true
    n112 = call <vilib>:"WPI_DashboardRetrieveStatusInfo.vi"("Binding Refnum"=w185, "Window Mode Notifier"=w182, "TCP Cnx"="TCP") -> ("Power and Errors"=w186:T17, "Robot Metrics"=w189:T18, "Status Info"=w190:T19, "Control Info"=w187:T20, "Robot Mode"=w184:T4, "Process?"=w188:bool)  [unwired: 3 in]
    "Mode" <- w184
    n113 = case shown="True" w188 {
      tunnel: w190 -> [_ w248]
      tunnel: w189 -> [_ w247]
      tunnel: w187 -> [_ w246]
      tunnel: w186 -> [_ w245]
      tunnel: w184 -> [_ _]
      frame False {
        n114 = Wait (ms)(milliseconds to wait=u32 20) -> ()  [unwired: 1 out]
      }
      frame True {
        # "swap motors to match\ncharts and include battery"
        n115 = Unbundle By Name(w246) -> ("Joystick Values"=w236:T21)  [unwired: 1 out]
        n116 = Unbundle By Name(w248) -> ()  [unwired: 2 out]
        n117 = Unbundle By Name(w247) -> ()  [unwired: 1 out]
        n118 = Unbundle By Name(w245) -> ("Robot IP"=→"Robot IP":string)
        n119 = call-poly <vilib>:"NT Write Value.vi"("Numeric"="Degrees Rotated", "Name"="Degree") -> ()  [unwired: 9 in, 1 out]
        n120 = call-poly <vilib>:"NT Write Value.vi"("Numeric"="NumAcq", "Name"="NumAcq") -> ()  [unwired: 9 in, 1 out]
        n121 = case shown="\"1\", Default" "Station" {
          frame "1", Default {
            n122 = call-poly <vilib>:"NT Write Value.vi"("String"="1", "Name"="Station Over") -> ()  [unwired: 9 in, 1 out]
          }
          frame "2" {
            n123 = call-poly <vilib>:"NT Write Value.vi"("String"="2", "Name"="Station Over") -> ()  [unwired: 9 in, 1 out]
          }
          frame "3" {
            n124 = call-poly <vilib>:"NT Write Value.vi"("String"="3", "Name"="Station Over") -> ()  [unwired: 9 in, 1 out]
          }
        }
        n125 = Index Array(array=w236) -> (element #1=w235:T22, element #3=w221:T22)  [unwired: 4 in, 2 out]
        n126 = call-poly <vilib>:"NT Write Value.vi"("Boolean"="OVERRIDE", "Name"="Override") -> ()  [unwired: 9 in, 1 out]
        n127 = call-poly <vilib>:"NT Write Value.vi"("Numeric"="Forward Time", "Name"="DriveForTime") -> ()  [unwired: 9 in, 1 out]
        n128 = call-poly <vilib>:"NT Read Value.vi"("Name"="Vision Error") -> ("Numeric"=→"Error Value":dbl)  [unwired: 9 in, 1 out]
        n129 = call-poly <vilib>:"NT Write Value.vi"("Boolean"="Comp Bot?", "Name"="WhichBot") -> ()  [unwired: 9 in, 1 out]
        n130 = call-poly <vilib>:"NT Write Value.vi"("Boolean"="Left Station", "Name"="Left Station") -> ()  [unwired: 9 in, 1 out]
        n131 = call "Prepare Joystick Data for Displays.vi"("Joystick Values"=w235) -> ("Buttons"=→"JS1 Buttons":T23, "Z Axis"=→"JS1 Z":dbl, "Cartesian Data"=→"JS1 Graph":cluster{"X axis":dbl, "X axis":dbl}[])  [unwired: 8 in]
        n132 = call "Prepare Joystick Data for Displays.vi"("Joystick Values"=w221) -> ("Buttons"=→"JS2 Buttons":T23, "Z Axis"=→"JS2 Z":dbl, "Cartesian Data"=→"JS2 Graph":cluster{"X axis":dbl, "X axis":dbl}[])  [unwired: 8 in]
        n133 = call-poly <vilib>:"NT Write Value.vi"("Numeric"="Offset", "Name"="Offset Value") -> ()  [unwired: 9 in, 1 out]
        n134 = call-poly <vilib>:"NT Write Value.vi"("Numeric"="Target Drive Speed", "Name"="DrivSpeed") -> ()  [unwired: 9 in, 1 out]
        n135 = call-poly <vilib>:"NT Write Value.vi"("Numeric"="Degree  Error", "Name"="DegErr") -> ()  [unwired: 9 in, 1 out]
        n136 = call-poly <vilib>:"NT Read Value.vi"("Name"="RobotDrive Motors") -> ("Numeric Array"=w227:dbl[])  [unwired: 9 in, 1 out]
        n137 = call-poly <vilib>:"NT Read Value.vi"("Name"="Gyro") -> ("Numeric"=w224:dbl)  [unwired: 9 in, 1 out]
        n138 = call-poly <vilib>:"NT Write Value.vi"("Numeric"="Acq Boundary", "Name"="Boundary") -> ()  [unwired: 9 in, 1 out]
        n139 = call-poly <vilib>:"NT Write Value.vi"("Numeric"="Target Pivot Speed", "Name"="PivSpeed") -> ()  [unwired: 9 in, 1 out]
        n140 = Quotient & Remainder(x=w224, y=360.0) -> (x-y*floor(x/y)=→"Gyro":dbl)  [unwired: 1 out]
        n141 = Index Array(array=w227, index #1=1, index #4=0) -> (element #1=w240:dbl, element #2=w241:dbl, element #3=w239:dbl, element #4=w244:dbl)  [unwired: 2 in]
        n142 = call-poly <vilib>:"NT Write Value.vi"("Boolean"="New Gyro", "Name"="Gyro") -> ()  [unwired: 9 in, 1 out]
        n143 = Bundle("Numeric"=w239, "Numeric"=w240) -> (→"MotorChart R" →"MotorSliders R":cluster{"Numeric":dbl, "Numeric":dbl})  [unwired: 1 in]
        n144 = Bundle("Numeric"=w241, "Numeric"=w244) -> (→"MotorChart L" →"MotorSliders L":cluster{"Numeric":dbl, "Numeric":dbl})  [unwired: 1 in]
      }
    }
  }
  n145 = while {
    tunnel: [w264] -> _
    tunnel: w73 -> [w263]
    tunnel: w69 -> [w262]
    tunnel: w68 -> [w261]
    tunnel: w67 -> [_]
    tunnel: w63 -> [w260]
    tunnel: w28 -> [w259]
    tunnel: w26 -> [w258]
    shift-right: [w257] -> _
    shift-left: _ -> [w256]
    tunnel: w20 -> [w255]
    i -> [w264]
    stop <- FALSE stop-if-true
    n146 = event shown="[0] Timeout" {
      selector: w261 -> [_ _ _ _ _ _ _ _ _ _ _ _ _ _ _ _ _ _ _ _ _]
      dyn-events: [_ _ _ _ _ _ _ _ _ _ _ _ _ _ _ _ w520 _ _ _ _] -> _
      timeout: u32 60 ("milliseconds to wait") -> [_ _ _ _ _ _ _ _ _ _ _ _ _ _ _ _ _ _ _ _ _]
      tunnel: w263 -> [w276 _ _ _ _ _ _ _ _ _ _ _ _ _ _ _ _ _ _ _ _]
      tunnel: "Test Tree" -> [_ _ _ _ _ _ _ _ _ _ _ w487 w495 w497 w501 w509 _ _ _ _ _]
      tunnel: w262 -> [_ _ _ _ _ _ _ _ _ _ _ _ _ _ _ _ w522 _ w540 _ _]
      tunnel: w260 -> [_ _ _ _ _ _ _ _ _ _ _ _ _ _ _ _ w518 _ _ _ _]
      tunnel: w259 -> [_ _ _ _ _ _ _ _ _ _ _ _ _ _ _ _ w514 _ _ _ _]
      tunnel: w258 -> [w271 _ _ _ _ _ w438 _ _ _ _ _ _ _ _ _ _ _ _ _ _]
      tunnel: [w270 w315 w417 w422 w431 w435 w436 w445 w455 w462 w474 w486 w493 w496 w500 w508 w513 w535 w537 w541 w552] -> w257
      tunnel: w256 -> [w270 w315 w417 w422 w431 w435 w436 _ _ w462 w474 w486 w493 w496 w500 w508 w513 w535 w537 w541 w552]
      tunnel: w255 -> [w268 _ _ _ _ _ _ _ _ _ _ _ _ _ _ _ _ _ _ _ _]
      event Timeout {
        n147 = event-data() -> ()  [unwired: 1 in, 1 out]
        n148 = call <vilib>:"Connextion Info.vi"() -> ("Connected"=→"NT Connection":bool)  [unwired: 10 in, 1 out]
        n149 = local read "Mode"() -> (w273:T4)
        n150 = case shown="\"Test\"" "Dashboard Tab" {
          tunnel: w276 -> [_ _ w292 _ _]
          tunnel: "/TestMode/Automatic/" ("Name Pattern") -> [_ _ w291 _ _]
          tunnel: T24 [{"Operation"=enum."Clear", "Color Box"=14013909}, {"Operation"=enum."Clear", "Color Box"=14013909}, {"Operation"=enum."Clear", "Color Box"=14013909}, {"Operation"=enum."Clear", "Color Box"=14013909}, {"Operation"=enum."Update", "Color Box"=14013909}, {"Operation"=enum."Update", "Color Box"=16777215}, {"Operation"=enum."Clear", "Color Box"=14013909}, {"Operation"=enum."Clear", "Color Box"=14013909}, {"Operation"=enum."Clear", "Color Box"=14013909}] -> [_ _ w284 _ w308]
          tunnel: w273 -> [_ _ w283 _ w307]
          tunnel: u32[] [15790320, 15790320, 15790320, 15790320, 16777215, 16777215, 15790320, 15790320, 15790320] -> [_ _ _ _ w313]
          tunnel: w271 -> [_ _ _ _ w301]
          tunnel: w268 -> [_ w278 _ _ _]
          frame "Custom", Default {
          }
          frame "Basic" {
            n151 = call <vilib>:"WPI_DashboardUpdateNames.vi"("Controls on Tab"=w278) -> ()  [unwired: 11 in]
          }
          frame "Test" {
            w290 = -2 ("Active Item:Row Number")
            n152 = Index Array(array=w284, index=w283) -> (element=w285:T27)
            n153 = Unbundle(w285) -> ("Operation"=w286:enum16{"Update", "Clear"}, "Color Box"=w287:u32)
            n154 = call <vilib>:"NT Read and Format Entries as Tree.vi"("Operation"=w286, "Name Pattern"=w291, "Tree Refnum"=w292) -> ()  [unwired: 7 in, 2 out]
            n155 = call <vilib>:"NT Read String.vi"("Name"="/TestMode/TestName") -> ("String"=w281:string)  [unwired: 9 in, 1 out]
            n156 = case shown="\"\"" w281 {
              tunnel: "/TestMode/TestProgress" ("Name") -> [w294 _]
              tunnel: "/TestMode/TestProgressText" ("Name") -> [w293 _]
              frame Default {
                n157 = call <vilib>:"NT Read Number.vi"("Name"=w294) -> ("Numeric"=w295:dbl)  [unwired: 9 in, 1 out]
                n158 = call <vilib>:"NT Read String.vi"("Name"=w293) -> ("String"=w296:string)  [unwired: 9 in, 1 out]
                n159 = Bundle("Numeric"=w295, "String"=w296) -> (→"Progress":cluster{"Numeric":dbl, "String":string})  [unwired: 1 in]
              }
              frame "" {
                n160 = local write "Test Name"(u16 0) -> ()
                n161 = property on="Progress" class="Clust (strict)"("Visible"=FALSE) -> ()  [unwired: 2 in, 2 out]
              }
            }
            n162 = property on="Test Tree" class="Tree (strict)"("Active Item Row Number"=w290, "ActiveColNum"=w290, "CellBG"=w287, "Active Item Row Number"=-1 ("Active Item:Row Number"), "CellBG"=u32 5789784 ("Color Box")) -> ()  [unwired: 2 in, 2 out]
          }
          frame "Variables" {
            n163 = control-ref of="Tree"() -> (w300:refnum<vi>)
            n164 = call <vilib>:"NT Read and Format Entries as Tree.vi"("Tree Refnum"=w300) -> ()  [unwired: 9 in, 2 out]
          }
          frame "Commands" {
            w309 = u32 5789784 ("Color Box")
            w310 = T28 {"Row"=-1, "Column"=-2} ("Active Cell:Active Cell")
            w312 = T28 {"Row"=-2, "Column"=-2} ("Active Cell:Active Cell")
            n165 = Index Array(array=w308, index=w307) -> (element=w306:T27)
            n166 = Index Array(array=w313, index=w307) -> (element=w311:u32)
            n167 = local read "Command Selection"() -> (w304:i32)
            n168 = property on="Command Selection" class="MCListbox (strict)"("ActiveCell"=w312, "CellBG"=w311, "ActiveCell"=w310, "CellBG"=w309) -> ()  [unwired: 2 in, 2 out]
            n169 = property on="Command Params" class="Tbl (strict)"("Active Cell"=w312, "Cell BG Color"=w311, "Active Cell"=w310, "Cell BG Color"=w309) -> ()  [unwired: 2 in, 2 out]
            n170 = Unbundle(w306) -> ("Operation"=w305:enum16{"Update", "Clear"})  [unwired: 1 out]
            n171 = call <vilib>:"WPI_DashboardUpdate RPC Info.vi"("Operation"=w305) -> ("update"=w303:bool, "commands"=w302:string[][])  [unwired: 9 in]
            n172 = call <vilib>:"WPI_DashboardUpdate Command Params.vi"("Update"=w303, "NewVal"=w304, "Commands"=w302, "Param Tbl"=w301) -> ()  [unwired: 7 in, 1 out]
            n173 = property on="Command Selection" class="MCListbox (strict)"("ItemNames"=w302) -> ()  [unwired: 2 in, 2 out]
          }
        }
      }
      event "Test Tree": Value Change {
        # "Show appropriate\ncontrols"
        n174 = event-data() -> ("CtlRef"=w318:refnum<vi>, "NewVal"=w316:string)  [unwired: 1 in]
        n175 = call <vilib>:"WPI_UtilitiesGetTreeIOName.vi"("NewVal"=w316, "TreeControl in"=w318) -> ("I/O Name"=w319:string)  [unwired: 9 in]
        n176 = property on="Progress" class="Clust (strict)"("Visible"=FALSE) -> ()  [unwired: 2 in, 2 out]
        n177 = case shown="\"Camera\"" w319 {
          selector: w319 -> [_ w326 _ w348 w357 _]
          tunnel: w316 -> [_ _ w345 w347 _ w364]
          tunnel: cluster{string[]}[] [{["640x480", "320x240", "160x120"]}, {["Auto", "Fixed indoor", "Fixed outdoor 1", "Fixed outdoor 2", "Fixed fluorescent 1", "Fixed fluorescent 2", "Hold current"]}, {["Auto", "Flicker-free 50 Hz", "Flicker-free 60 Hz", "Hold current"]}, {["None", "Prioritize frame rate", "Prioritize image quality"]}, {["Monochrome", "Color"]}] -> [_ _ _ _ _ w363]
          frame Default {
            w321 = FALSE ("Visible")
            w320 = FALSE ("Visible")
            n178 = property on="Test Slider" class="Slide (strict)"("Visible"=w321) -> ()  [unwired: 2 in, 2 out]
            n179 = property on="On/Off" class="Bool (strict)"("Visible"=w321) -> ()  [unwired: 2 in, 2 out]
            n180 = property on="Rev/Fwd" class="Clust (strict)"("Visible"=w321) -> ()  [unwired: 2 in, 2 out]
            n181 = property on="Test Ring" class="Ring (strict)"("Visible"=w320) -> ()  [unwired: 2 in, 2 out]
            n182 = property on="Motor" class="Clust (strict)"("Visible"=w320) -> ()  [unwired: 2 in, 2 out]
          }
          frame "Analog Out", "Motor", "PWM" {
            w327 = FALSE ("Visible")
            n183 = case shown="\"Analog Out\"" w326 {
              tunnel: [1.0 ("Value") -1.0 ("Value") 0.0 ("Value")] -> w325
              tunnel: [255.0 ("Value") 1.0 ("Value") 5.0 ("Value")] -> w324
              tunnel: [128.0 ("Value") 0.0 ("Value") 0.0 ("Value")] -> w323
              tunnel: [64.0 ("Value") 0.5 ("Value") 1.0 ("Value")] -> w322
              frame "PWM" {
              }
              frame "Motor", Default {
              }
              frame "Analog Out" {
              }
            }
            n184 = property on="Test Slider" class="Slide (strict)"("Visible"=w327) -> ()  [unwired: 2 in, 2 out]
            n185 = property on="Test Ring" class="Ring (strict)"("Visible"=w327) -> ()  [unwired: 2 in, 2 out]
            n186 = property on="On/Off" class="Bool (strict)"("Visible"=w327) -> ()  [unwired: 2 in, 2 out]
            n187 = property on="Rev/Fwd" class="Clust (strict)"("Visible"=w327) -> ()  [unwired: 2 in, 2 out]
            n188 = property on="Motor" class="Clust (strict)"("Visible"=TRUE) -> ()  [unwired: 2 in, 2 out]
            n189 = property on="Value" class="Slide (strict)"("Value"=w323, "Scale.Minimum"=w325, "Scale.Maximum"=w324, "Scale.Increment"=w322) -> ()  [unwired: 2 in, 2 out]
          }
          frame "Servo" {
            w343 = FALSE ("Visible")
            n190 = call <vilib>:"NT Read Number.vi"("Name"=w345) -> ("Numeric"=w344:dbl)  [unwired: 9 in, 1 out]
            n191 = property on="Motor" class="Clust (strict)"("Visible"=w343) -> ()  [unwired: 2 in, 2 out]
            n192 = property on="Test Ring" class="Ring (strict)"("Visible"=w343) -> ()  [unwired: 2 in, 2 out]
            n193 = property on="On/Off" class="Bool (strict)"("Visible"=w343) -> ()  [unwired: 2 in, 2 out]
            n194 = property on="Rev/Fwd" class="Clust (strict)"("Visible"=w343) -> ()  [unwired: 2 in, 2 out]
            n195 = property on="Test Slider" class="Slide (strict)"("Visible"=TRUE, "Scale.Maximum"=170.0 ("Scale.Range:Maximum")) -> ()  [unwired: 2 in, 2 out]
            n196 = local write "Test Slider"(w344) -> ()
          }
          frame "Relay", "Solenoid" {
            w346 = FALSE ("Visible")
            n197 = property on="Motor" class="Clust (strict)"("Visible"=w346) -> ()  [unwired: 2 in, 2 out]
            n198 = property on="Test Slider" class="Slide (strict)"("Visible"=w346) -> ()  [unwired: 2 in, 2 out]
            n199 = property on="Test Ring" class="Ring (strict)"("Visible"=w346) -> ()  [unwired: 2 in, 2 out]
            n200 = Search and Replace String(input string=w347, search string="/Value  **", replace string="/Direction") -> (result string=w353:string)  [unwired: 5 in, 3 out]
            n201 = call <vilib>:"NT Read String.vi"("Name"=w353) -> ("String"=w351:string)  [unwired: 9 in, 1 out]
            n202 = Equal?(x="Both directions", y=w351) -> (x = y?=w349:bool)
            n203 = property on="Rev/Fwd" class="Clust (strict)"("Visible"=w349) -> ()  [unwired: 2 in, 2 out]
            n204 = Not(x=w349) -> (.not. x?=w350:bool)
            n205 = property on="On/Off" class="Bool (strict)"("Visible"=w350, "Caption.Text"=w348) -> ()  [unwired: 2 in, 2 out]
          }
          frame "Compressor", "Digital Out" {
            w356 = FALSE ("Visible")
            # "Get direction and finish"
            n206 = property on="Test Ring" class="Ring (strict)"("Visible"=w356) -> ()  [unwired: 2 in, 2 out]
            n207 = property on="Motor" class="Clust (strict)"("Visible"=w356) -> ()  [unwired: 2 in, 2 out]
            n208 = property on="Test Slider" class="Slide (strict)"("Visible"=w356) -> ()  [unwired: 2 in, 2 out]
            n209 = property on="Rev/Fwd" class="Clust (strict)"("Visible"=FALSE) -> ()  [unwired: 2 in, 2 out]
            n210 = property on="On/Off" class="Bool (strict)"("Visible"=TRUE, "Caption.Text"=w357) -> ()  [unwired: 2 in, 2 out]
          }
          frame "Camera" {
            n211 = call <vilib>:"Get Last Path Segment.vi"("String in"=w364) -> ("String out"=w365:string)  [unwired: 10 in]
            n212 = property on="On/Off" class="Bool (strict)"("Visible"=FALSE) -> ()  [unwired: 2 in, 2 out]
            n213 = case shown="\"White Balance  **\"" w365 {
              tunnel: w364 -> [w371 w380 w389 w398 w407 _ w413]
              tunnel: w363 -> [w369 w377 w386 w395 w404 _ _]
              frame "Size  **" {
                n214 = Index Array(array=w369) -> (element=w368:cluster{string[]})  [unwired: 1 in]
                n215 = call <vilib>:"NT Read String.vi"("Name"=w371) -> ("String"=w370:string)  [unwired: 9 in, 1 out]
                n216 = property on="Test Slider" class="Slide (strict)"("Visible"=FALSE) -> ()  [unwired: 2 in, 2 out]
                n217 = property on="Test Ring" class="Ring (strict)"("Visible"=TRUE) -> ()  [unwired: 2 in, 2 out]
                n218 = Unbundle(w368) -> (w366:string[])
                n219 = Match First String(2:w366, 3:w370) -> (0:w367:i32)  [unwired: 1 out]
                n220 = property on="Test Ring" class="Ring (strict)"("Value"=w367, "Strings []"=w366) -> ()  [unwired: 2 in, 2 out]
              }
              frame "White Balance  **" {
                n221 = call <vilib>:"NT Read String.vi"("Name"=w380) -> ("String"=w379:string)  [unwired: 9 in, 1 out]
                n222 = Index Array(array=w377, index=1) -> (element=w378:cluster{string[]})
                n223 = property on="Test Slider" class="Slide (strict)"("Visible"=FALSE) -> ()  [unwired: 2 in, 2 out]
                n224 = property on="Test Ring" class="Ring (strict)"("Visible"=TRUE) -> ()  [unwired: 2 in, 2 out]
                n225 = Unbundle(w378) -> (w375:string[])
                n226 = Match First String(2:w375, 3:w379) -> (0:w374:i32)  [unwired: 1 out]
                n227 = property on="Test Ring" class="Ring (strict)"("Value"=w374, "Strings []"=w375) -> ()  [unwired: 2 in, 2 out]
              }
              frame "Exposure  **" {
                n228 = call <vilib>:"NT Read String.vi"("Name"=w389) -> ("String"=w388:string)  [unwired: 9 in, 1 out]
                n229 = Index Array(array=w386, index=2) -> (element=w387:cluster{string[]})
                n230 = property on="Test Slider" class="Slide (strict)"("Visible"=FALSE) -> ()  [unwired: 2 in, 2 out]
                n231 = property on="Test Ring" class="Ring (strict)"("Visible"=TRUE) -> ()  [unwired: 2 in, 2 out]
                n232 = Unbundle(w387) -> (w383:string[])
                n233 = Match First String(2:w383, 3:w388) -> (0:w384:i32)  [unwired: 1 out]
                n234 = property on="Test Ring" class="Ring (strict)"("Value"=w384, "Strings []"=w383) -> ()  [unwired: 2 in, 2 out]
              }
              frame "Exposure Priority  **" {
                n235 = call <vilib>:"NT Read String.vi"("Name"=w398) -> ("String"=w397:string)  [unwired: 9 in, 1 out]
                n236 = Index Array(array=w395, index=3) -> (element=w396:cluster{string[]})
                n237 = property on="Test Slider" class="Slide (strict)"("Visible"=FALSE) -> ()  [unwired: 2 in, 2 out]
                n238 = property on="Test Ring" class="Ring (strict)"("Visible"=TRUE) -> ()  [unwired: 2 in, 2 out]
                n239 = Unbundle(w396) -> (w392:string[])
                n240 = Match First String(2:w392, 3:w397) -> (0:w393:i32)  [unwired: 1 out]
                n241 = property on="Test Ring" class="Ring (strict)"("Value"=w393, "Strings []"=w392) -> ()  [unwired: 2 in, 2 out]
              }
              frame "Color Enable  **" {
                n242 = call <vilib>:"NT Read String.vi"("Name"=w407) -> ("String"=w406:string)  [unwired: 9 in, 1 out]
                n243 = Index Array(array=w404, index=4) -> (element=w405:cluster{string[]})
                n244 = property on="Test Slider" class="Slide (strict)"("Visible"=FALSE) -> ()  [unwired: 2 in, 2 out]
                n245 = property on="Test Ring" class="Ring (strict)"("Visible"=TRUE) -> ()  [unwired: 2 in, 2 out]
                n246 = Unbundle(w405) -> (w401:string[])
                n247 = Match First String(2:w401, 3:w406) -> (0:w402:i32)  [unwired: 1 out]
                n248 = property on="Test Ring" class="Ring (strict)"("Value"=w402, "Strings []"=w401) -> ()  [unwired: 2 in, 2 out]
              }
              frame Default {
                n249 = property on="Test Slider" class="Slide (strict)"("Visible"=FALSE) -> ()  [unwired: 2 in, 2 out]
                n250 = property on="Test Ring" class="Ring (strict)"("Visible"=FALSE) -> ()  [unwired: 2 in, 2 out]
              }
              frame "Brightness  **", "Color Level  **", "Compression  **", "FPS  **", "Sharpness  **" {
                n251 = call <vilib>:"NT Read Number.vi"("Name"=w413) -> ("Numeric"=w412:dbl)  [unwired: 9 in, 1 out]
                n252 = property on="Test Ring" class="Ring (strict)"("Visible"=FALSE) -> ()  [unwired: 2 in, 2 out]
                n253 = property on="Test Slider" class="Slide (strict)"("Visible"=TRUE, "Scale.Maximum"=100.0 ("Scale.Range:Maximum")) -> ()  [unwired: 2 in, 2 out]
                n254 = local write "Test Slider"(w412) -> ()
              }
            }
            n255 = property on="Motor" class="Clust (strict)"("Visible"=FALSE) -> ()  [unwired: 2 in, 2 out]
            n256 = property on="Rev/Fwd" class="Clust (strict)"("Visible"=FALSE) -> ()  [unwired: 2 in, 2 out]
          }
        }
      }
      event "Test Name": Mouse Enter {
        # "Populate the ring with the list of tests"
        n257 = event-data() -> ()  [unwired: 1 in, 1 out]
        n258 = call <vilib>:"NT Read String Array.vi"("Name"="/TestMode/TestList") -> ("String Array"=w421:string[])  [unwired: 9 in, 1 out]
        n259 = Build Array (concatenate)("Select the test to run...", w421) -> (w420:string[])
        n260 = property on="Test Name" class="Ring (strict)"("Strings []"=w420) -> ()  [unwired: 2 in, 2 out]
      }
      event "Test Name": Value Change {
        w423 = FALSE ("Visible")
        # "Tell the robot the test name to run"
        n261 = event-data() -> ("NewVal"=w427:u16)  [unwired: 1 in]
        n262 = property on="Test Name" class="Ring (strict)"() -> ("Strings []"=w428:string[])  [unwired: 2 in, 2 out]
        n263 = property on="Test Ring" class="Ring (strict)"("Visible"=w423) -> ()  [unwired: 2 in, 2 out]
        n264 = property on="Motor" class="Clust (strict)"("Visible"=w423) -> ()  [unwired: 2 in, 2 out]
        n265 = property on="Test Slider" class="Slide (strict)"("Visible"=w423) -> ()  [unwired: 2 in, 2 out]
        n266 = property on="On/Off" class="Bool (strict)"("Visible"=w423) -> ()  [unwired: 2 in, 2 out]
        n267 = property on="Rev/Fwd" class="Clust (strict)"("Visible"=w423) -> ()  [unwired: 2 in, 2 out]
        n268 = local write "Progress"(T6 {"Test Progress"=0, "Test Progress Text"=""} ("Progress")) -> ()
        n269 = property on="Progress" class="Clust (strict)"("Visible"=TRUE) -> ()  [unwired: 2 in, 2 out]
        n270 = Index Array(array=w428, index=w427) -> (element=w426:string)
        n271 = call <vilib>:"NT Write String.vi"("String"=w426, "Name"="/TestMode/TestName") -> ()  [unwired: 9 in, 1 out]
      }
      event "Select Auto": Mouse Enter {
        # "Populate the combo box with the list of autonomous options"
        n272 = event-data() -> ()  [unwired: 1 in, 1 out]
        n273 = call <vilib>:"NT Read String Array.vi"("Name"="Auto List") -> ("String Array"=w430:string[])  [unwired: 9 in, 1 out]
        n274 = property on="Select Auto" class="CmbBox"("Strings[]"=w430) -> ()  [unwired: 2 in, 2 out]
      }
      event "Select Auto": Value Change {
        # "User modified the Auto Selection. Write to NT variable so robot knows."
        n275 = event-data() -> ("NewVal"=w433:string)  [unwired: 1 in]
        n276 = call <vilib>:"NT Write String.vi"("String"=w433, "Name"="Auto Selector") -> ()  [unwired: 9 in, 1 out]
      }
      event "Command Selection": Value Change {
        # "Get the params and show in table"
        n277 = event-data() -> ("NewVal"=w439:i32)  [unwired: 1 in]
        n278 = property on="Command Selection" class="MCListbox (strict)"() -> ("ItemNames"=w437:string[][])  [unwired: 2 in, 2 out]
        n279 = call <vilib>:"WPI_DashboardUpdate Command Params.vi"("NewVal"=w439, "Commands"=w437, "Param Tbl"=w438) -> ()  [unwired: 8 in, 1 out]
      }
      event "Execute Command": Value Change {
        # "Started one, Unique ID holds\nresponse"
        n280 = event-data() -> ()  [unwired: 1 in, 1 out]
        n281 = property on="Command Selection" class="MCListbox (strict)"() -> ("ItemNames"=w450:string[][])  [unwired: 2 in, 2 out]
        n282 = Index Array(array=w450, index (row)="Command Selection", index (col)=0) -> (element=w448:string)
        n283 = call <vilib>:"Invoke Commands.vi"("Command Params"="Command Params", "Function Name"=w448) -> ("Params"=w444:u8, "Started"=w443:bool)  [unwired: 7 in, 1 out]
        n284 = Array Subset(array="Command Params", length (row)=w444) -> (w445:string[][])  [unwired: 3 in]
        n285 = Select(t="Executing" ("Cmd Status"), s=w443, f="" ("Cmd Status")) -> (s? t:f=→"Cmd Status":string)
      }
      event "Command Selection": Double Click {
        n286 = event-data() -> ("Row"=w458:i32)  [unwired: 1 in]
        n287 = property on="Command Selection" class="MCListbox (strict)"() -> ("ItemNames"=w461:string[][])  [unwired: 2 in, 2 out]
        n288 = local read "Command Params"() -> (w457:string[][])
        n289 = Index Array(array=w461, index (row)=w458, index (col)=0) -> (element=w459:string)
        n290 = call <vilib>:"Invoke Commands.vi"("Command Params"=w457, "Function Name"=w459) -> ("Params"=w456:u8, "Started"=w451:bool)  [unwired: 7 in, 1 out]
        n291 = Array Subset(array=w457, length (row)=w456) -> (w455:string[][])  [unwired: 3 in]
        n292 = Select(t="Executing" ("Cmd Status"), s=w451, f="" ("Cmd Status")) -> (s? t:f=w452:string)
        n293 = local write "Cmd Status"(w452) -> ()
      }
      event "CheckList": Double Click {
        # "Shift clears all"
        # "Update symbols on the listbox"
        n294 = event-data() -> ("PlatMods.Shift"=w463:bool, "Row"=w465:i32)  [unwired: 1 in]
        n295 = case shown="True" w463 {
          tunnel: w465 -> [w469 _]
          tunnel: 1 -> [w468 _]
          frame False {
            n296 = property on="CheckList" class="LstBox (strict)"() -> ("Item Symbols"=w467:i32[])  [unwired: 2 in, 2 out]
            n297 = Replace Array Subset(array=w467, new element=w468, index=w469) -> (w466:i32[])
            n298 = property on="CheckList" class="LstBox (strict)"("Item Symbols"=w466) -> ()  [unwired: 2 in, 2 out]
          }
          frame True {
            w470 = 0 ("Top Row")
            n299 = property on="CheckList" class="LstBox (strict)"() -> ("Number of Rows"=w472:u32)  [unwired: 2 in, 2 out]
            n300 = Initialize Array(0, w472) -> (w471:i32[])
            n301 = property on="CheckList" class="LstBox (strict)"("Top Row"=w470, "Value"=w470, "Item Symbols"=w471) -> ()  [unwired: 2 in, 2 out]
          }
        }
      }
      event "CheckList": Key Down {
        # "Update symbols on the listbox\nLeft and right keys check and uncheck"
        n302 = event-data() -> ("VKey"=w476:T25)  [unwired: 1 in]
        n303 = case shown="\"Left\", \"Right\"" w476 {
          selector: w476 -> [w481 _]
          tunnel: eventvkey."Left" ("VKey") -> [w479 _]
          frame "Left", "Right" {
            n304 = Equal?(x=w479, y=w481) -> (x = y?=w480:bool)
            n305 = Select(t=0, s=w480, f=1) -> (s? t:f=w482:i32)
            n306 = property on="CheckList" class="LstBox (strict)"() -> ("Item Symbols"=w485:i32[])  [unwired: 2 in, 2 out]
            n307 = Replace Array Subset(array=w485, new element=w482, index="CheckList") -> (w484:i32[])
            n308 = property on="CheckList" class="LstBox (strict)"("Item Symbols"=w484) -> ()  [unwired: 2 in, 2 out]
          }
          frame Default {
          }
        }
      }
      event "Motor.Enable": Value Change {
        # "When the test mode otor enable helper is set, update that\ntree row item's value"
        n309 = event-data() -> ("NewVal"=w491:bool)  [unwired: 1 in]
        n310 = Unbundle("Motor") -> ("Value"=w490:dbl)  [unwired: 1 out]
        n311 = Select(t=w490, s=w491, f=0.0) -> (s? t:f=w488:dbl)
        n312 = call <vilib>:"NT Write Number.vi"("Numeric"=w488, "Name"=w487) -> ()  [unwired: 9 in, 1 out]
      }
      event "Test Slider": Value Change {
        # "When the test mode slider helper is set, update that\ntree row item's value"
        n313 = event-data() -> ("NewVal"=w494:dbl)  [unwired: 1 in]
        n314 = call <vilib>:"NT Write Number.vi"("Numeric"=w494, "Name"=w495) -> ()  [unwired: 9 in, 1 out]
      }
      event "On/Off": Value Change {
        # "When the test mode on/off helper value is set, update that\ntree row item's value"
        n315 = event-data() -> ("NewVal"=w499:bool)  [unwired: 1 in]
        n316 = Boolean To (0,1)(Boolean=w499) -> (0, 1=w498:i16)
        n317 = call <vilib>:"NT Write Number.vi"("Numeric"=w498, "Name"=w497) -> ()  [unwired: 9 in, 1 out]
      }
      event "Rev/Fwd": Value Change {
        # "When the test mode helper value for relays is set, update that\ntree row item's value"
        n318 = event-data() -> ("NewVal.Forward"=w507:bool, "NewVal.Reverse"=w506:bool)  [unwired: 1 in]
        n319 = Boolean To (0,1)(Boolean=w507) -> (0, 1=w503:i16)
        n320 = Boolean To (0,1)(Boolean=w506) -> (0, 1=w505:i16)
        n321 = Negate(x=w505) -> (-x=w504:i16)
        n322 = Add(x=w503, y=w504) -> (x+y=w502:i16)
        n323 = call <vilib>:"NT Write Number.vi"("Numeric"=w502, "Name"=w501) -> ()  [unwired: 9 in, 1 out]
      }
      event "Test Ring": Value Change {
        # "When a test mode helper value is selected from the ring,\nset the tree item's variable to the string value"
        n324 = event-data() -> ("NewVal"=w511:u16)  [unwired: 1 in]
        n325 = property on="Test Ring" class="Ring (strict)"() -> ("Strings []"=w512:string[])  [unwired: 2 in, 2 out]
        n326 = Index Array(array=w512, index=w511) -> (element=w510:string)
        n327 = call <vilib>:"NT Write String.vi"("String"=w510, "Name"=w509) -> ()  [unwired: 9 in, 1 out]
      }
      event "Rec Mode": Value Change {
        # "Update globals for recording mode and path to read log from.\nClear when logging and let NetworkTables set path for vision to\nuse."
        n328 = event-data() -> ("NewVal"=w523:enum32{"Stop", "Record", "Playback"})  [unwired: 1 in]
        n329 = global write "WPI_DashboardLogging Global.vi" "Recording"(w523) -> ()
        n330 = global write "WPI_DashboardLogging Global.vi" "Logging Filename"(path "") -> ()
        n331 = case shown="\"Playback\"" w523 {
          tunnel: w522 -> [_ w525 w534]
          tunnel: [_ _ w533] -> w520
          tunnel: [_ _ w532] -> _
          tunnel: w518 -> [_ _ w530]
          tunnel: cluster{i32, i32} {-250, 170} -> [_ _ w529]
          tunnel: [_ _ T26 {"Image Size"=TRUE, "Image Type"=TRUE, "Pixel Value"=TRUE, "ROI Information"=TRUE, "Zoom Factor"=FALSE} ("Image Information Shown:All Elements")] -> w516
          tunnel: [_ _ TRUE ("Zoom Factor")] -> w515
          tunnel: w514 -> [_ _ w526]
          frame Default {
          }
          frame "Stop", "Record" {
            # "Place Window too"
            n332 = invoke class="VI" method="FP.Close"(reference=w525) -> (reference out=w524:refnum<vi>)  [unwired: 2 in, 2 out]
            n333 = invoke class="VI" method="Abort VI"(reference=w524) -> ()  [unwired: 2 in, 3 out]
          }
          frame "Playback" {
            n334 = call "Open Playback Panel.vi"("Offset"=w529, "DB VI Ref"=w530, "Playback in"=w534) -> ("Playback out"=w531:refnum<vi>)  [unwired: 8 in]
            n335 = register-events(w531, w526) -> (reference out=w533:refnum<event-registration>, error out=w532:errorcluster)  [unwired: 2 in]
          }
        }
        n336 = call <vilib>:"WPI_DashboardNT Log FieldName Cache.vi"("Operation"=enum16{"Lookup/Add", "Index", "Clear"}."Clear") -> ()  [unwired: 8 in, 3 out]
        n337 = property on="Camera Image" class="ImageControl"("Image Information Shown"=w516, "Image Information Visible"=w515) -> ()  [unwired: 2 in, 2 out]
      }
      event Panel Close {
        w536 = enum32{"Stop", "Record", "Playback"}."Stop" ("Rec Mode")
        # "Playback window has been closed, abort"
        n338 = event-data() -> ()  [unwired: 1 in, 4 out]
        n339 = local write "Rec Mode"(w536) -> ()
        n340 = global write "WPI_DashboardLogging Global.vi" "Recording"(w536) -> ()
      }
      event Panel Close {
        # "Abort playback window and ourself"
        n341 = event-data() -> ()  [unwired: 1 in, 4 out]
        n342 = invoke class="VI" method="FP.Close"(reference=w540) -> (reference out=w539:refnum<vi>)  [unwired: 2 in, 2 out]
        n343 = invoke class="VI" method="Abort VI"(reference=w539) -> (error out=w538:errorcluster)  [unwired: 2 in, 2 out]
        n344 = invoke class="VI" method="Abort VI"(error in=w538) -> ()  [unwired: 2 in, 3 out]
      }
      event User Event {
        n345 = event-data() -> ("IDs"=w547:cluster{"RPC field ID":u16, "Unique ID":u16}, "String"=w546:string)  [unwired: 1 in]
        n346 = Bundle("IDs"=w547, "String"=w546) -> (w545:T8)  [unwired: 1 in]
        n347 = local write "Cmd Status"("" ("Cmd Status")) -> ()
        n348 = call <vilib>:"Retrieve RPC Response.vi"("RPC Response"=w545) -> ("Output"=w543:string[][])  [unwired: 10 in]
        n349 = Build Array (concatenate)(w541, w543) -> (w542:string[][])
        n350 = local write "Command Params"(w542) -> ()
      }
      event "Tree": Double Click {
        n351 = event-data() -> ("PlatMods"=w551:T29, "Tag"=w550:string)  [unwired: 1 in]
        n352 = Unbundle(w551) -> ("Shift"=w549:bool)  [unwired: 4 out]
        n353 = Not(x=w549) -> (.not. x?=w548:bool)
        n354 = call <vilib>:"NT Update Persistence.vi"("Persistence"=w548, "Name"=w550) -> ()  [unwired: 9 in, 1 out]
      }
    }
  }
  n355 = call "Adjust Dashboard Window.vi"("Sizing Refnums"=w51, "Size Constraints"=w55, "VI"=w63, "WIn Mode"=w37) -> ()  [unwired: 8 in]
  n356 = while {
    tunnel: w60 -> [w564]
    tunnel: w38 -> [w562]
    tunnel: [w560] -> _
    tunnel: u32 1000 ("milliseconds to wait") -> [w559]
    tunnel: w28 -> [w553]
    i -> [w560]
    stop <- FALSE stop-if-true
    n357 = Wait on Notification(notifier=w562, timeout in ms (-1)=w559) -> (notification=w561:string, timed out?=w557:bool)  [unwired: 2 in, 2 out]
    n358 = local read "Rec Mode"() -> (w555:enum32{"Stop", "Record", "Playback"})
    n359 = Equal?(x=w555, y=u16 2 ("Rec Mode")) -> (x = y?=w556:bool)
    n360 = Compound Arithmetic op=OR(invert w557, w556) -> (w558:bool)
    n361 = case shown="True" w558 {
      tunnel: w564 -> [_ w567]
      tunnel: w561 -> [_ w566]
      tunnel: w553 -> [_ w565]
      frame False {
      }
      frame True {
        n362 = call <vilib>:"Bind Controls to SmartDashboard.vi"("RPC ref"=w565, "Bound Control Refs"=w567, "Server IP Address"=w566) -> ()  [unwired: 9 in]
      }
    }
  }
